vi "MB Mater-Eth_RegisterWRITE.vi"() -> ()   [LabVIEW 2014]
uses:
  Program Files/National Instruments/LabVIEW 2014/nimodbus121/86/vi.lib/NI Modbus.llb/MB Modbus Command.ctl
panel:
  in  "Modbus Command":T1={"Function Code"=16, "Starting Address"=10, "Quantity"=2, "Data"=[], "Discrete"=[]} {"Function Code" items=["Read Coils"=1, "Read Discrete Inputs"=2, "Read Holding Registers"=3, "Read Input Registers"=4, "Write Single Coil"=5, "Write Single Register"=6, "Read Exception Status"=7, "Write Multiple Coils"=15, "Write Multiple Registers"=16]}
  in  "Array":u16[](array[numeric])
  in  "stop":bool
  in  "Remote Port 2":u16=502
  in  "Remote IP Address 2":string="127.0.0.1"
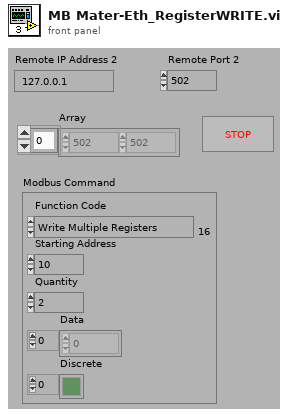
[diagram p1: front panel]
types:
  T1 = typedef "MB Modbus Command.ctl" = cluster{"Function Code":u8, "Starting Address":u16, "Quantity":u16, "Data":u16[], "Discrete":bool[]}
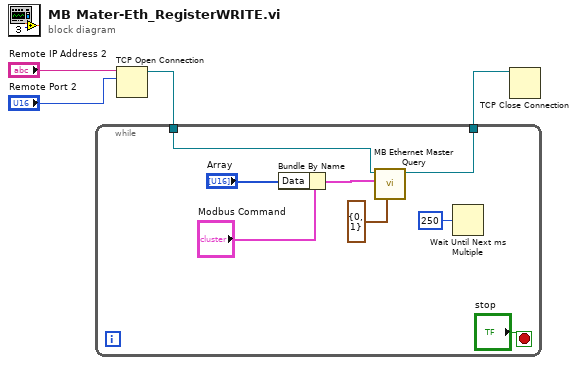
[diagram p0: block diagram]
diagram:
  n1 = TCP Open Connection(address="Remote IP Address 2", remote port or service name="Remote Port 2") -> (connection ID=w2:refnum<k5>)  [unwired: 3 in, 1 out]
  n2 = while {
    tunnel: w2 -> [w9]
    tunnel: [w8] -> w1
    stop <- "stop" stop-if-true
    n3 = Bundle By Name(cluster="Modbus Command", "Data"="Array") -> (w10:T1)
    n4 = call "MB Ethernet Master Query.vi"("MBAP Header"=cluster{"Transaction ID":u16, "Unit ID":u8} {"Transaction ID"=0, "Unit ID"=1}, "Modbus Command"=w10, "TCP Connection Refnum in"=w9) -> ("TCP Connection Refnum (dup)"=w8:refnum<k5>)  [unwired: 4 in, 4 out]
    n5 = Wait Until Next ms Multiple(millisecond multiple=u32 250) -> ()  [unwired: 1 out]
  }
  n6 = TCP Close Connection(connection ID=w1) -> ()  [unwired: 2 in, 2 out]
